vi "FPGA Read All FIFO Address by Name.vi"(8 "error in (no error)":errorcluster, 9 "Name":string, 11 "FPGA Interface Base in":refnum<class "FPGA Interface Base.lvclass">) -> (0 "error out":errorcluster, 1 "Found?":bool, 2 "Address":u32, 3 "FPGA Interface Base out":refnum<class "FPGA Interface Base.lvclass">)   [LabVIEW 2010, in "FPGA Interface Base.lvclass"]
uses:
  <userlib>/_FPGA Interface Advanced Tools/FPGA Interface Base/FPGA Interface Base.lvclass
  <userlib>/_FPGA Interface Advanced Tools/FPGA Interface Base/FPGA Interface Base.lvclass/FPGA Interface Base.ctl
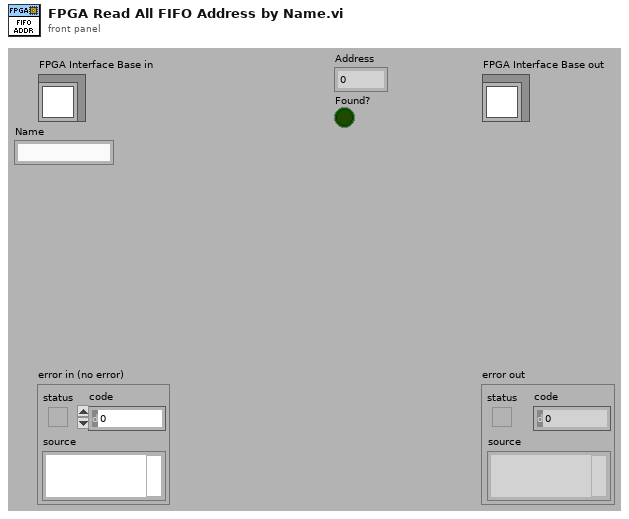
[diagram p1: front panel]
types:
  T1 = typedef "FPGA Interface Base.lvclass/FPGA Session.ctl" = refnum<data-value>
  T2 = typedef "FPGA Interface Base.lvclass/FPGA Session Data.ctl" = cluster{"Session Out":u32, "Indicator Scalars":T3, "Indicator Arrays":T5, "Control Scalars":T3, "Control Arrays":T5, "TargetToHost FIFO Channels":T7, "HostToTarget FIFO Channels":T7, "All FIFOs":T8[], "IRQ Context Queue":refnum<queue>}
  T3 = typedef "FPGA Bitfile Utility.lvlib/Scalar Register Set.ctl" = cluster{"Boolean":T4[], "I8":T4[], "I16":T4[], "I32":T4[], "I64":T4[], "U8":T4[], "U16":T4[], "U32":T4[], "U64":T4[]}
  T4 = typedef "FPGA Bitfile Utility.lvlib/Scalar Register.ctl" = cluster{"Address":u32, "Name":string}
  T5 = typedef "FPGA Bitfile Utility.lvlib/Array Register Set.ctl" = cluster{"Boolean":T6[], "I8":T6[], "I16":T6[], "I32":T6[], "I64":T6[], "U8":T6[], "U16":T6[], "U32":T6[], "U64":T6[]}
  T6 = typedef "FPGA Bitfile Utility.lvlib/Array Register.ctl" = cluster{"Address":u32, "Num Elements":u32, "Name":string}
  T7 = typedef "FPGA Bitfile Utility.lvlib/FIFO Channel Set.ctl" = cluster{"Boolean":T8[], "I8":T8[], "I16":T8[], "I32":T8[], "I64":T8[], "U8":T8[], "U16":T8[], "U32":T8[], "U64":T8[]}
  T8 = typedef "FPGA Bitfile Utility.lvlib/FIFO Channel.ctl" = cluster{"Physical Channel":u32, "Name":string}
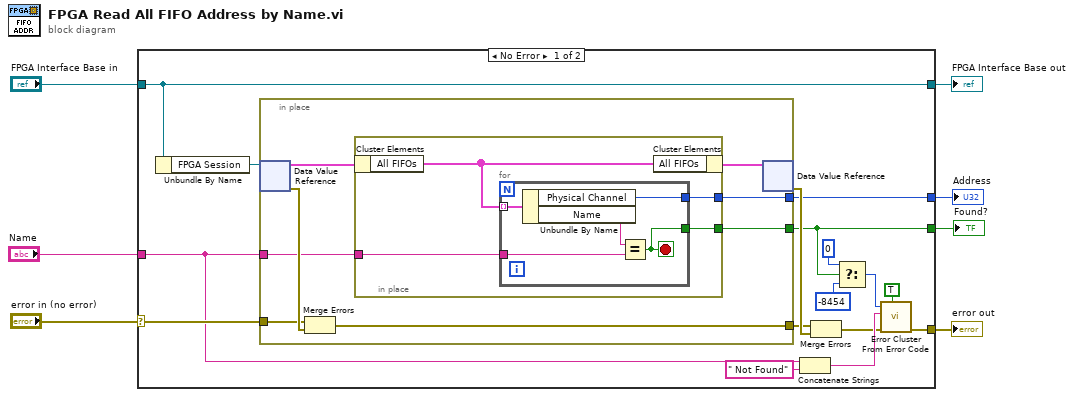
[diagram p0: block diagram]
diagram:
  n1 = case shown="No Error" "error in (no error)" {
    selector: "error in (no error)" -> [w18 w41]
    tunnel: [w11 w41] -> w6
    tunnel: [w23 w42] -> w4
    tunnel: "FPGA Interface Base in" -> [w23 w42]
    tunnel: [w19 _] -> w3
    tunnel: [w8 _] -> w2
    tunnel: "Name" -> [w9 _]
    frame No Error {
      n2 = Unbundle By Name(w23) -> ("FPGA Session"=w20:T1)
      n3 = in-place {
        in-place-border: w9 -> [w28]
        in-place-border: [w27] -> w19
        in-place-border: [w26] -> w8
        in-place-border: [w25] -> w21
        in-place-border: w18 -> [w24]
        n4 = in-place-dvr #1(w20) -> (w30:T2, w31:errorcluster)
        n5 = Merge Errors(w24, w31) -> (w25:errorcluster)
        n6 = in-place {
          in-place-border: w28 -> [w34]
          in-place-border: [w33] -> w27
          in-place-border: [w32] -> w26
          n7 = in-place-cluster #2(w30) -> ("All FIFOs"=w35:T8[])
          n8 = for {
            tunnel: w35 -> [w40] mode=indexing
            tunnel: [w38] -> w33
            tunnel: [w37] -> w32
            tunnel: w34 -> [w36]
            stop <- w37 stop-if-true
            n9 = Unbundle By Name(w40) -> ("Physical Channel"=w38:u32, "Name"=w39:string)
            n10 = Equal?(x=w39, y=w36) -> (x = y?=w37:bool)
          }
          n11 = in-place-cluster #2("All FIFOs"=w35) -> (w29:T2)
        }
        n12 = in-place-dvr #1(w29) -> (w22:errorcluster)  [unwired: 1 out]
      }
      n13 = Concatenate Strings(w9, " Not Found" ("string")) -> (w17:string)
      n14 = Merge Errors(w21, w22) -> (w10:errorcluster)
      n15 = Select(t=0, s=w8, f=-8454 ("error code (0)")) -> (s? t:f=w12:i32)
      n16 = call <vilib>:"Error Cluster From Error Code.vi"("show call chain? (False)"=TRUE, "error in (no error)"=w10, "error message (\"\")"=w17, "error code (0)"=w12) -> ("error out"=w11:errorcluster)  [unwired: 5 in]
    }
    frame Error {
    }
  }
  "error out" <- w6
  "FPGA Interface Base out" <- w4
  "Address" <- w3
  "Found?" <- w2
